vi "Update-GUI-values.vi"(8 "error in (no error)":errorcluster, 10 "New values":T1(array[cluster]), 11 "Controls in":refnum<vi>[](array[refnum])) -> (0 "error out":errorcluster, 1 "Values/controls match?":bool, 3 "Controls out":refnum<vi>[](array[refnum]))   [LabVIEW 2013, in "SettingsFile.lvlib" / "SettingsFile.lvclass"]
uses:
  SettingsFile.lvclass
  Messages.ctl
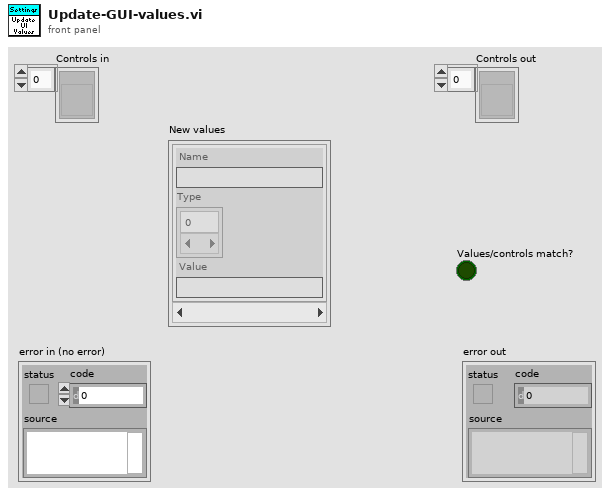
[diagram p1: front panel]
types:
  T1 = cluster{"Name":string, "Type":i16[], "Value":string}[]
  T2 = typedef "SettingsFile.lvlib/SettingsFile.lvclass/Messages.ctl" = enum16{"Time out", "User cancel", "Module cancel", "File format change"}
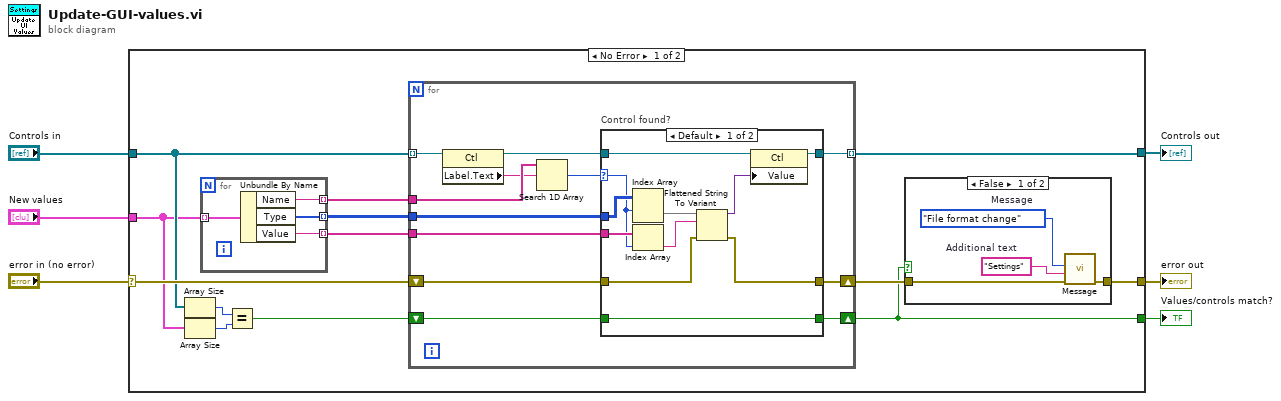
[diagram p0: block diagram]
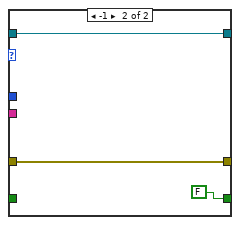
[diagram p3: hidden frame]
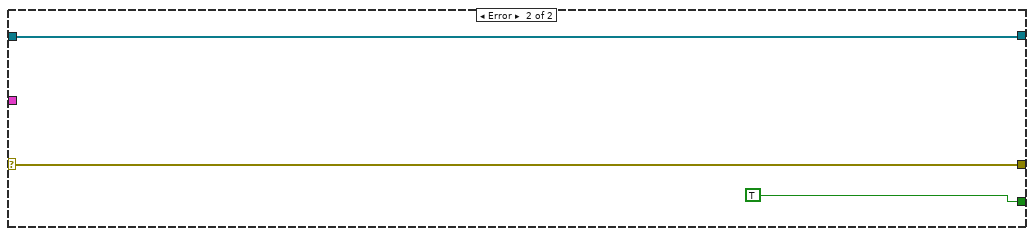
[diagram p4: hidden frame]
diagram:
  n1 = case shown="No Error" "error in (no error)" {
    selector: "error in (no error)" -> [w19 w57]
    tunnel: [w7 w57] -> w5
    tunnel: "Controls in" -> [w15 w56]
    tunnel: [w10 w56] -> w3
    tunnel: "New values" -> [w14 _]
    tunnel: [w8 TRUE] -> w1
    frame No Error {
      n2 = Array Size(array=w15) -> (size(s)=w13:i32)
      n3 = Array Size(array=w14) -> (size(s)=w12:i32)
      n4 = for {
        tunnel: w14 -> [w28] mode=indexing
        tunnel: [w27] -> w18 mode=indexing
        tunnel: [w26] -> w17 mode=indexing
        tunnel: [w25] -> w16 mode=indexing
        n5 = Unbundle By Name(w28) -> ("Name"=w27:string, "Type"=w26:i16[], "Value"=w25:string)
      }
      n6 = Equal?(x=w13, y=w12) -> (x = y?=w11:bool)
      n7 = for {
        tunnel: w15 -> [w40] mode=indexing
        shift-right: [w30] -> w9
        shift-left: w19 -> [w31]
        tunnel: w18 -> [w39]
        tunnel: w17 -> [w32]
        tunnel: w16 -> [w33]
        shift-right: [w36] -> w8
        shift-left: w11 -> [w37]
        tunnel: [w29] -> w10 mode=indexing
        n8 = property class="Ctl"(reference=w40) -> (reference out=w34:refnum<vi>, "Label.Text"=w38:string)  [unwired: 1 in, 1 out]
        n9 = Search 1D Array(1D array=w39, element=w38) -> (index of element=w35:i32)  [unwired: 1 in]
        n10 = case "Control found?" shown="Default" w35 {
          selector: w35 -> [w48 _]
          tunnel: w37 -> [w42 _]
          tunnel: [w42 FALSE] -> w36
          tunnel: w34 -> [w51 w52]
          tunnel: w33 -> [w49 _]
          tunnel: w32 -> [w50 _]
          tunnel: w31 -> [w45 w54]
          tunnel: [w44 w54] -> w30
          tunnel: [w41 w52] -> w29
          frame Default {
            n11 = Index Array(array=w50, index (row)=w48) -> (element=w47:i16[])  [unwired: 1 in]
            n12 = Index Array(array=w49, index=w48) -> (element=w46:string)
            n13 = Flattened String To Variant(4:w45, 6:w46, 7:w47) -> (0:w44:errorcluster, 3:w43:variant)
            n14 = property class="Ctl"(reference=w51, "Value"=w43) -> (reference out=w41:refnum<vi>)  [unwired: 1 in, 1 out]
          }
          frame -1 {
          }
        }
      }
      n15 = case shown="False" w8 {
        tunnel: w9 -> [w23 w24]
        tunnel: [w22 w24] -> w7
        frame False {
          w20 = "Settings"  # Additional text
          w21 = Messages."File format change"  # Message
          n16 = call "Message.vi"("error in (no error)"=w23, "Additional text"=w20, "Message"=w21) -> ("error out"=w22:errorcluster)  [unwired: 8 in]
        }
        frame True {
        }
      }
    }
    frame Error {
    }
  }
  "error out" <- w5
  "Controls out" <- w3
  "Values/controls match?" <- w1
